vi "Translation3d_RotateBy.vi"(10 "other Rot3d":T1={"Q_quaternion"={"R"=1.0, "V"=[0.0, 0.0, 0.0]}}, 11 "in Translation3D":T3 {"Z" format="%14.3f"; "Y" format="%14.3f"; "X" format="%14.3f"}) -> (3 "out Translation3d":T3 {"Z" format="%14.3f"; "Y" format="%14.3f"; "X" format="%14.3f"})   [LabVIEW 2019, in "Trajectory_Library.lvlib"]
doc: "Constructs a Translation2d with the provided distance and angle. This is essentially converting from polar coordinates to Cartesian coordinates.\n\nRepresents a translation in 2d space. This object can be used to represent a point or a vector.\n\nThis assumes that you are using conventional mathematical axes. When the robot is placed on the origin, facing toward the X direction, moving forward increases the X, whereas moving to the left increases the Y.\n\nParameters:\n - Dist - Distance.\n - Ang - Rotation representing the angle.\n\nReturns\n - TRANSLATION - The TRANSLATION data structure"
uses:
  Trajectory_Library.lvlib
  TRANSLATION3D.ctl
  ROTATION3D.ctl
  QUATERNION.ctl
  Quaternion_Get_LVQuat.vi
  Quaternion_New_LVQuat.vi
  Quaternion_Equals.vi
  <vilib>/robotics/Kinematics/Multiply Quaternions.vi
  <vilib>/robotics/Kinematics/Multiply Quaternion by Quaternion.vi
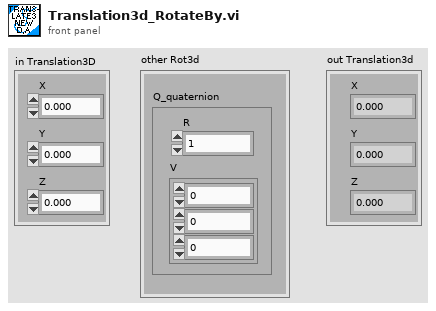
[diagram p1: front panel]
types:
  T1 = typedef "Trajectory_Library.lvlib/ROTATION3D.ctl" = cluster{"Q_quaternion":T2}
  T2 = typedef "Trajectory_Library.lvlib/QUATERNION.ctl" = cluster{"R":dbl, "V":dbl[]}
  T3 = typedef "Trajectory_Library.lvlib/TRANSLATION3D.ctl" = cluster{"X":dbl, "Y":dbl, "Z":dbl}
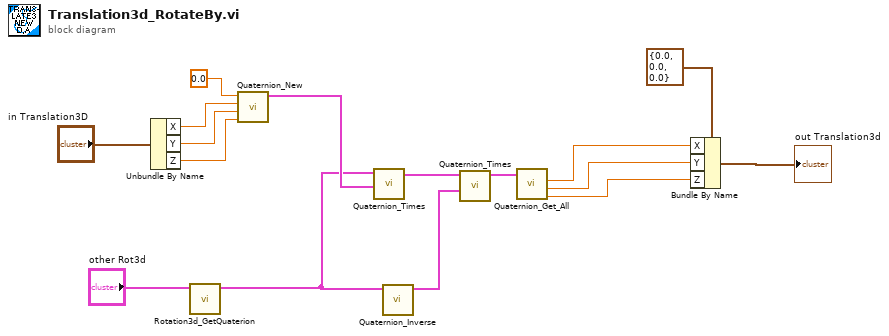
[diagram p0: block diagram]
diagram:
  n1 = Unbundle By Name("in Translation3D") -> ("X"=w13:dbl, "Y"=w12:dbl, "Z"=w11:dbl)
  n2 = call "Rotation3d_GetQuaterion.vi"("in Rotation3d"="other Rot3d") -> ("out Quaterion"=w9:T2)  [unwired: 10 in]
  n3 = call "Quaternion_New.vi"("Z"=w11, "Y"=w12, "X"=w13, "W"=0.0) -> ("out Quaternion"=w10:T2)  [unwired: 7 in]
  n4 = call "Quaternion_Times.vi"("Other Quaternion"=w10, "Quaternion"=w9) -> ("Times"=w8:T2)  [unwired: 9 in]
  n5 = call "Quaternion_Inverse.vi"("Quaternion"=w9) -> ("Inverse"=w7:T2)  [unwired: 10 in]
  n6 = call "Quaternion_Times.vi"("Other Quaternion"=w7, "Quaternion"=w8) -> ("Times"=w4:T2)  [unwired: 9 in]
  n7 = call "Quaternion_Get_All.vi"("Quaternion"=w4) -> ("Z"=w1:dbl, "Y"=w2:dbl, "X"=w3:dbl)  [unwired: 7 in, 1 out]
  n8 = Bundle By Name(cluster=T3 {"X"=0.0, "Y"=0.0, "Z"=0.0} ("TRANSLATION"), "X"=w3, "Y"=w2, "Z"=w1) -> (→"out Translation3d":T3)
